vi "Symphony Server test read.vi"() -> ()   [LabVIEW 2012]
panel:
  out "timed out":bool
  in  "Boolean":bool
  out "data":T1
  out "RemCom 2":bool
  out "ServerConn 2":refnum<k13>
  out "RemCom":bool
  out "ServerConn":refnum<k13>
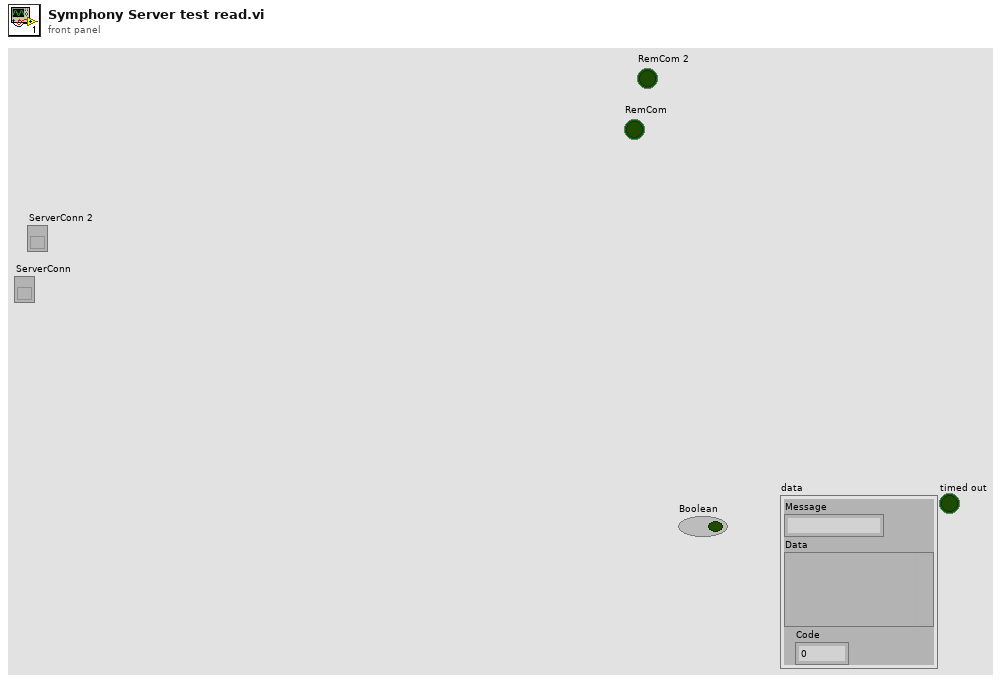
[diagram p1: front panel]
types:
  T1 = cluster{"Message":string, "Data":variant, "Code":i32}
  T2 = enum16{"Read", "Write", "ReadWrite", "BufferedRead", "BufferedReadWrite"}
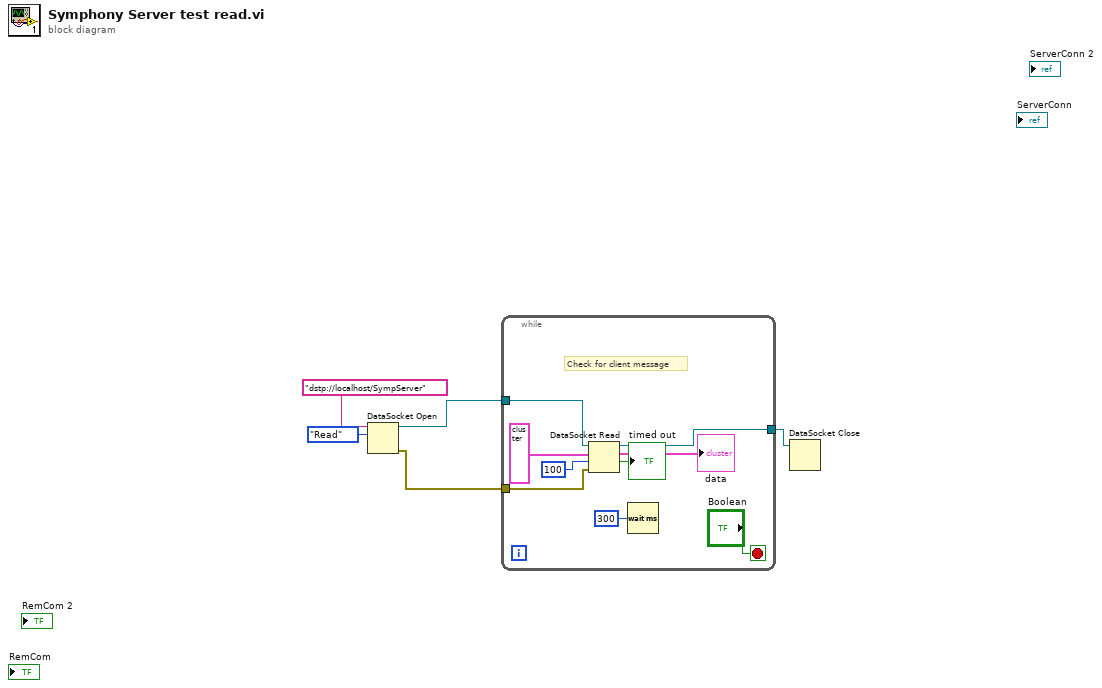
[diagram p0: block diagram]
diagram:
  n1 = DataSocket Open(10:T2."Read" ("mode"), 11:"dstp://localhost/SympServer" ("URL")) -> (0:w3:errorcluster, 3:w2:refnum<k13>)  [unwired: 2 in]
  n2 = while {
    tunnel: w3 -> [w14]
    tunnel: w2 -> [w13]
    tunnel: [w8] -> w1
    stop <- "Boolean" stop-if-true
    # "Check for client message"
    n3 = DataSocket Read(8:w14, 9:100 ("ms timeout (10000)"), 10:T1 {"Message"="", "Data"=variant, "Code"=0} ("SympClient"), 11:w13) -> (1:→"timed out":bool, 2:→"data":T1, 3:w8:refnum<k13>)  [unwired: 1 in, 4 out]
    n4 = Wait (ms)(milliseconds to wait=u32 300) -> ()  [unwired: 1 out]
  }
  n5 = DataSocket Close(11:w1) -> ()  [unwired: 2 in, 2 out]
